vi "Filter Particles.vi"(6 "Filter Settings":T1, 11 "Scores in":T2(array[cluster])) -> (1 "Rejected particles out":T2(array[cluster]), 3 "Good particles out":T2(array[cluster]))   [LabVIEW 2015]
uses:
  Particle Filter Settings.ctl
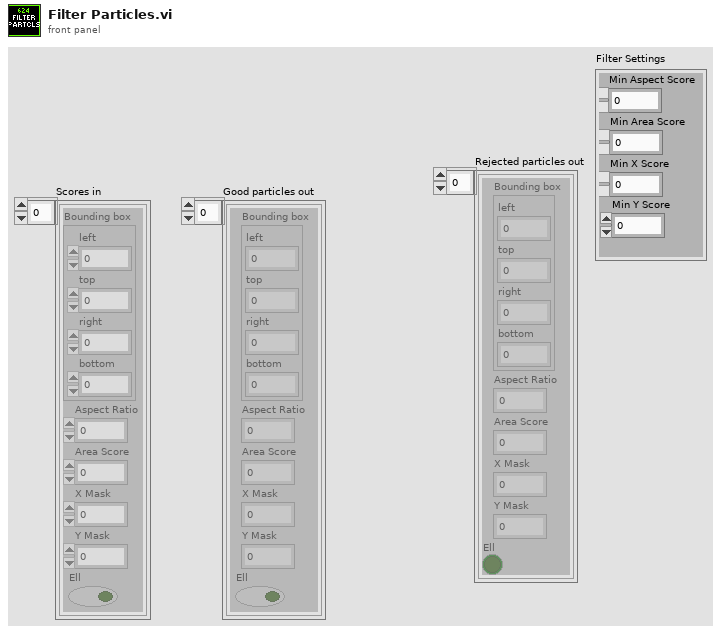
[diagram p1: front panel]
types:
  T1 = typedef "Particle Filter Settings.ctl" = cluster{"Min Aspect Score":dbl, "Min Area Score":dbl, "Min X Score":dbl, "Min Y Score":dbl}
  T2 = cluster{"Bounding box":cluster{"left":dbl, "top":dbl, "right":dbl, "bottom":dbl}, "Aspect Ratio":dbl, "Area Score":dbl, "X Mask":dbl, "Y Mask":dbl, "Ell":bool}[]
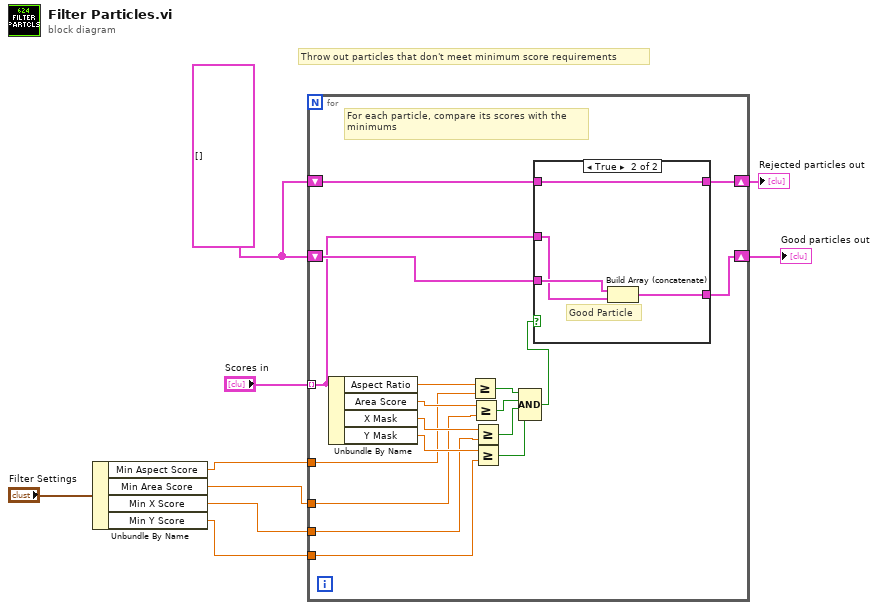
[diagram p0: block diagram]
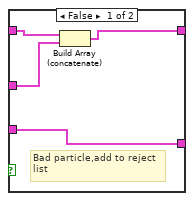
[diagram p2: hidden frame]
diagram:
  w7 = T2 [] ("Scores in")
  # "Throw out particles that don't meet minimum score requirements"
  n1 = Unbundle By Name("Filter Settings") -> ("Min Aspect Score"=w4:dbl, "Min Area Score"=w3:dbl, "Min X Score"=w2:dbl, "Min Y Score"=w1:dbl)
  n2 = for {
    tunnel: "Scores in" -> [w13] mode=indexing
    shift-right: [w12] -> w8
    shift-left: w7 -> [w14]
    tunnel: w4 -> [w23]
    tunnel: w3 -> [w22]
    tunnel: w2 -> [w21]
    tunnel: w1 -> [w20]
    shift-right: [w11] -> w6
    shift-left: w7 -> [w10]
    # "For each particle, compare its scores with the \nminimums"
    n3 = Unbundle By Name(w13) -> ("Aspect Ratio"=w27:dbl, "Area Score"=w26:dbl, "X Mask"=w25:dbl, "Y Mask"=w24:dbl)
    n4 = Greater Or Equal?(x=w27, y=w23) -> (x >= y?=w19:bool)
    n5 = Greater Or Equal?(x=w26, y=w22) -> (x >= y?=w18:bool)
    n6 = Greater Or Equal?(x=w25, y=w21) -> (x >= y?=w17:bool)
    n7 = Greater Or Equal?(x=w24, y=w20) -> (x >= y?=w16:bool)
    n8 = Compound Arithmetic op=AND(w19, w18, w17, w16) -> (w15:bool)
    n9 = case shown="True" w15 {
      tunnel: w14 -> [w31 w35]
      tunnel: w13 -> [w28 w33]
      tunnel: [w31 w34] -> w12
      tunnel: [w29 w32] -> w11
      tunnel: w10 -> [w30 w32]
      frame False {
        # "Bad particle,add to reject\nlist"
        n10 = Build Array (concatenate)(w30, w28) -> (w29:T2)
      }
      frame True {
        # "Good Particle"
        n11 = Build Array (concatenate)(w35, w33) -> (w34:T2)
      }
    }
  }
  "Good particles out" <- w8
  "Rejected particles out" <- w6
